vi "VoltageOutputStart.vi"(0 "Device Info":T1={"Serial Number"=-1, "Channel"=0, "Port"=0}, 5 "Voltage Output Range":i32(ring)=2 items=["VOLTAGE_OUTPUT_RANGE_10V"=1, "VOLTAGE_OUTPUT_RANGE_5V"=2], 7 "Enabled":bool=TRUE, 9 "Voltage":dbl, 11 "error in (no error)":errorcluster, 12 "Connection":u16(ring) items=["No Preference", "Remote", "Local"], 13 "Timeout (mSec)":i32=5000) -> (4 "Phidget ID":u64, 6 "Serial Number Return":i32, 10 "Attached?":bool, 15 "error out":errorcluster)   [LabVIEW 2020, in "Phidget Voltage Output.lvlib"]
doc: "${VoltageOutput:StartHeader}"
uses:
  <instrlib>/Phidgets/Phidget Voltage Output/Phidget Voltage Output.lvlib
  <instrlib>/Phidgets/Phidget Common/Phidget Common.lvlib
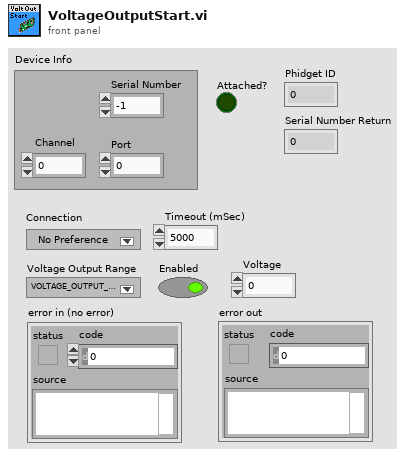
[diagram p1: front panel]
types:
  T1 = cluster{"Serial Number":i32, "Channel":i32, "Port":i32}
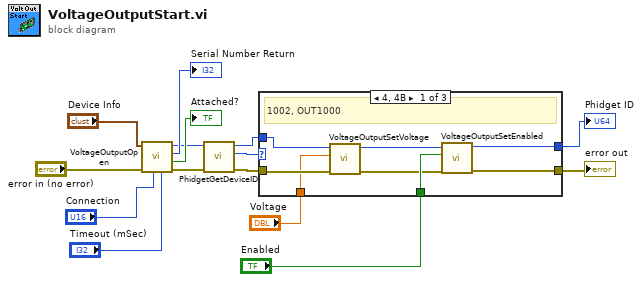
[diagram p0: block diagram]
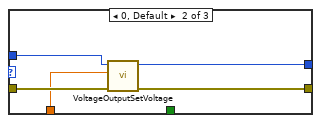
[diagram p2: hidden frame]
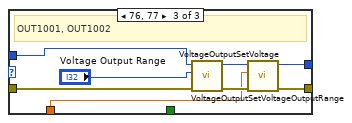
[diagram p3: hidden frame]
diagram:
  n1 = call <instrlib>:"VoltageOutputOpen.vi"("Timeout (mSec)"="Timeout (mSec)", "Connection"="Connection", "error in"="error in (no error)", "Device Info"="Device Info") -> ("error out"=w9:errorcluster, "Attached?"=→"Attached?":bool, "Serial Number Return"=→"Serial Number Return":i32, "Phidget ID"=w10:u64)  [unwired: 4 in]
  n2 = call <instrlib>:"PhidgetGetDeviceID.vi"("error in (no error)"=w9, "Device In"=w10) -> ("error out"=w6:errorcluster, "Devie IDs"=w8:u32, "Device Out"=w7:u64)  [unwired: 6 in]
  n3 = case shown="4, 4B" w8 {
    tunnel: w7 -> [w17 w28 w36]
    tunnel: w6 -> [w18 w27 w35]
    tunnel: [w23 w24 w30] -> w5
    tunnel: [w22 w25 w31] -> w4
    tunnel: "Enabled" -> [w21 _ _]
    tunnel: "Voltage" -> [w16 w26 w29]
    frame 4, 75 {
      # "1002, OUT1000"
      n4 = call <instrlib>:"VoltageOutputSetVoltage.vi"("error in (no error)"=w18, "Voltage"=w16, "Device In"=w17) -> ("error out"=w19:errorcluster, "Device Out"=w20:u64)  [unwired: 6 in]
      n5 = call <instrlib>:"VoltageOutputSetEnabled.vi"("error in (no error)"=w19, "Enabled"=w21, "Device In"=w20) -> ("error out"=w22:errorcluster, "Device Out"=w23:u64)  [unwired: 6 in]
    }
    frame 0, Default {
      n6 = call <instrlib>:"VoltageOutputSetVoltage.vi"("error in (no error)"=w27, "Voltage"=w26, "Device In"=w28) -> ("error out"=w25:errorcluster, "Device Out"=w24:u64)  [unwired: 6 in]
    }
    frame 76, 77 {
      # "OUT1001, OUT1002"
      n7 = call <instrlib>:"VoltageOutputSetVoltageOutputRange.vi"("error in (no error)"=w35, "Voltage Output Range"="Voltage Output Range", "Device In"=w36) -> ("error out"=w32:errorcluster, "Device Out"=w33:u64)  [unwired: 6 in]
      n8 = call <instrlib>:"VoltageOutputSetVoltage.vi"("error in (no error)"=w32, "Voltage"=w29, "Device In"=w33) -> ("error out"=w31:errorcluster, "Device Out"=w30:u64)  [unwired: 6 in]
    }
  }
  "error out" <- w4
  "Phidget ID" <- w5
